vi "Change Digits of Precision.vi"(6 "VI Path":path, 7 "Digits of Precision":u8, 8 "error in (no error)":errorcluster, 10 "Numeric Constant Name":string) -> (0 "error out":errorcluster)   [LabVIEW 2018]
doc: "Changes the digits of precision of a named floating point numeric constant on the block diagram of a vi"
uses:
  <vilib>/Utility/traverseref.llb/TRef TravTarget.ctl
  <vilib>/Utility/traverseref.llb/VI Scripting - Traverse.lvlib
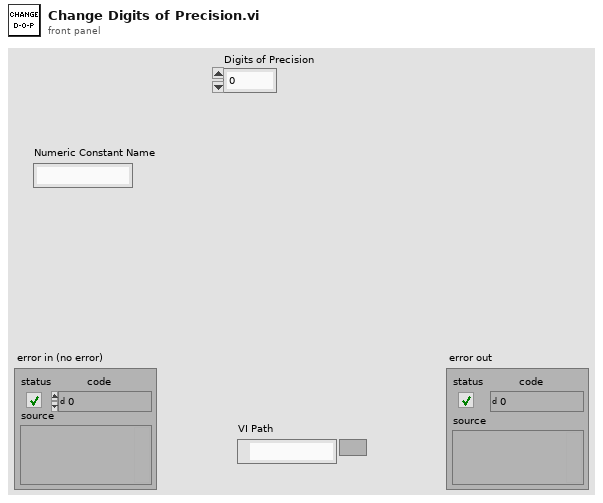
[diagram p1: front panel]
types:
  T1 = typedef "TRef TravTarget.ctl" = enum16{"FP", "BD", "Other"}
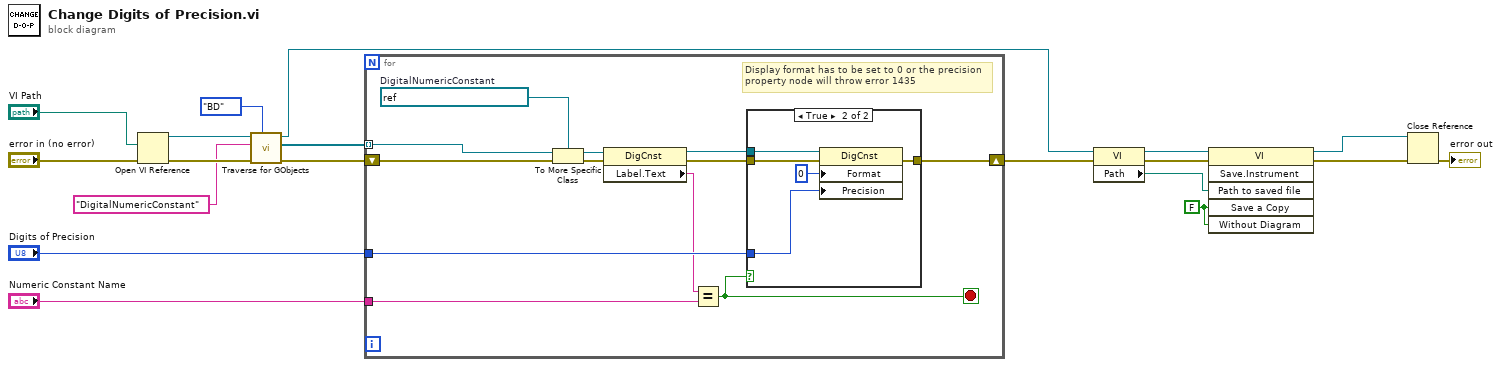
[diagram p0: block diagram]
diagram:
  w1 = FALSE ("Save a Copy")
  n1 = Open VI Reference(vi path="VI Path", error in (no error)="error in (no error)") -> (vi reference=w11:refnum<vi>, error out=w13:errorcluster)  [unwired: 4 in]
  n2 = call <vilib>:"Traverse for GObjects.vi"("Traverse Target"=TRef_TravTarget."BD", "error in (no error)"=w13, "Class Name"="DigitalNumericConstant", "VI Refnum"=w11) -> ("error out"=w12:errorcluster, "References"=w8:refnum<vi>[], "dup VI Refnum"=w4:refnum<vi>)  [unwired: 4 in, 1 out]
  n3 = for {
    tunnel: w8 -> [w31] mode=indexing
    shift-right: [w26] -> w17
    shift-left: w12 -> [w27]
    tunnel: "Numeric Constant Name" -> [w30]
    tunnel: "Digits of Precision" -> [w28]
    stop <- w29 stop-if-true
    w25 = refnum<vi> refnum  # DigitalNumericConstant
    # "Display format has to be set to 0 or the precision property node will throw error 1435"
    n4 = To More Specific Class(target class=w25, reference=w31, error in=w27) -> (specific class reference=w24:refnum<vi>, error out=w21:errorcluster)
    n5 = property class="DigCnst"(reference=w24, error in=w21) -> (reference out=w22:refnum<vi>, error out=w20:errorcluster, "Label.Text"=w23:string)
    n6 = Equal?(x=w23, y=w30) -> (x = y?=w29:bool)
    n7 = case shown="True" w29 {
      tunnel: w22 -> [_ w37]
      tunnel: w28 -> [_ w34]
      tunnel: w20 -> [w32 w36]
      tunnel: [w32 w35] -> w26
      frame False {
      }
      frame True {
        n8 = property class="DigCnst"(reference=w37, error in=w36, "Format"=u8 0 ("Display Format:Format"), "Precision"=w34) -> (error out=w35:errorcluster)  [unwired: 1 out]
      }
    }
  }
  n9 = property class="VI"(reference=w4, error in=w17) -> (reference out=w3:refnum<vi>, error out=w5:errorcluster, "Path"=w2:path)
  n10 = invoke class="VI" method="Save.Instrument"(reference=w3, error in=w5, "Path to saved file"=w2, "Save a Copy"=w1, "Without Diagram"=w1) -> (reference out=w6:refnum<vi>, error out=w7:errorcluster)  [unwired: 1 in, 4 out]
  n11 = Close Reference(reference=w6, error in (no error)=w7) -> (error out=→"error out":errorcluster)
